vi "CommandParser.vi"(0 "Settings in":T3, 5 "UART_Command":T2, 9 "Cmd_data":u16) -> (4 "Settings out":T3, 6 "UART Reply":T1, 10 "Reply_Data":u16)   [LabVIEW 2013, in "UART_Firmware.lvlib"]
uses:
  UART_Firmware.lvlib
  Settings.ctl
  Parity.ctl
  StopBits.ctl
  UART_Command.ctl
  UART_Response.ctl
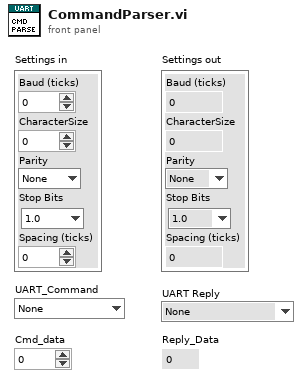
[diagram p1: front panel]
types:
  T1 = typedef "UART_Firmware.lvlib/UART_Response.ctl" = enum8{"None", "Rx", "BaudHighAck", "BaudLowAck", "CharSizeAck", "ParityAck", "StopBitsAck", "SpacingHighAck", "SpacingLowAck", "ParityError", "FrameError"}
  T2 = typedef "UART_Firmware.lvlib/UART_Command.ctl" = enum8{"None", "Tx", "SetBaud_High", "SetBaud_Low", "SetCharLength", "SetParity", "SetStopBits", "SetSpacing_High", "SetSpacing_Low"}
  T3 = typedef "UART_Firmware.lvlib/Settings.ctl" = cluster{"Baud (ticks)":u32, "CharacterSize":u8, "Parity":T4, "Stop Bits":T5, "Spacing (ticks)":u32}
  T4 = typedef "UART_Firmware.lvlib/Parity.ctl" = enum8{"None", "Even", "Odd"}
  T5 = typedef "UART_Firmware.lvlib/StopBits.ctl" = enum8{"1.0", "1.5", "2.0"}
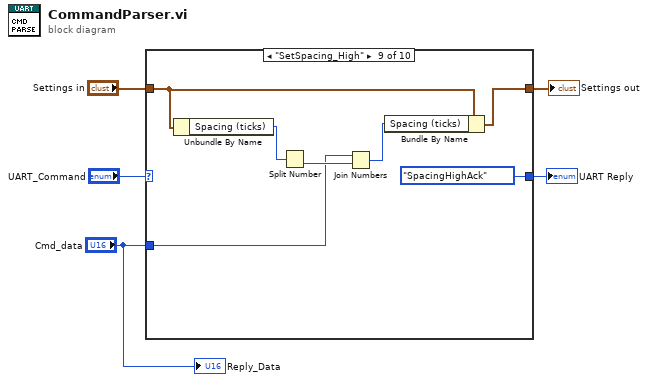
[diagram p0: block diagram]
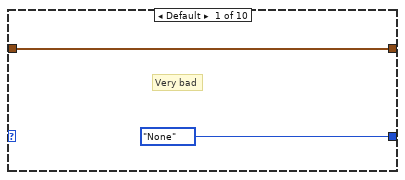
[diagram p2: hidden frame]
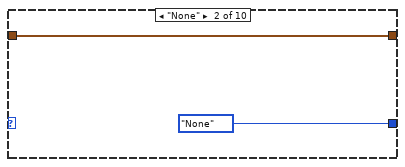
[diagram p3: hidden frame]
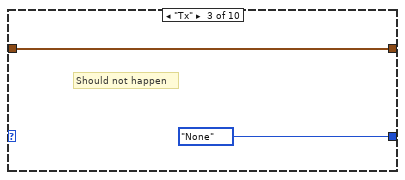
[diagram p4: hidden frame]
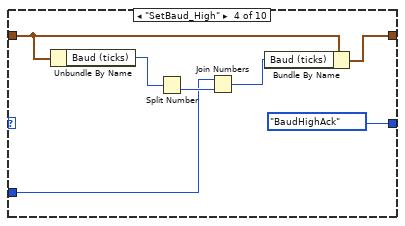
[diagram p5: hidden frame]
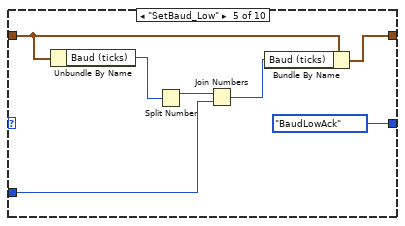
[diagram p6: hidden frame]
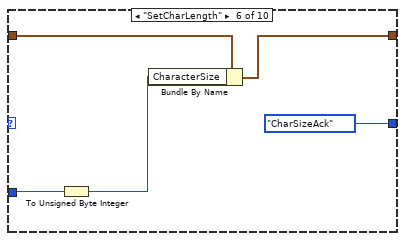
[diagram p7: hidden frame]
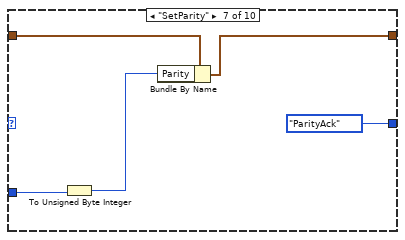
[diagram p8: hidden frame]
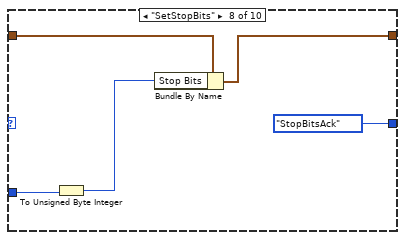
[diagram p9: hidden frame]
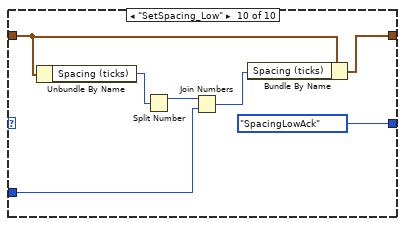
[diagram p10: hidden frame]
diagram:
  n1 = case shown="\"SetSpacing_High\"" "UART_Command" {
    tunnel: "Settings in" -> [w6 w9 w11 w18 w25 w30 w35 w40 w46 w53]
    tunnel: "Cmd_data" -> [_ _ _ w13 w20 w27 w32 w37 w41 w49]
    tunnel: [w6 w9 w11 w16 w23 w29 w34 w39 w47 w54] -> w3
    tunnel: [UART_Response."None" ("UART Reply") UART_Response."None" ("UART Reply") UART_Response."None" ("UART Reply") UART_Response."BaudHighAck" ("UART Reply") UART_Response."BaudLowAck" ("UART Reply") UART_Response."CharSizeAck" ("UART Reply") UART_Response."ParityAck" ("UART Reply") UART_Response."StopBitsAck" ("UART Reply") UART_Response."SpacingHighAck" ("UART Reply") UART_Response."SpacingLowAck" ("UART Reply")] -> w2
    frame Default {
      # "Very bad"
    }
    frame "None" {
    }
    frame "Tx" {
      # "Should not happen"
    }
    frame "SetBaud_High" {
      n2 = Unbundle By Name(w18) -> ("Baud (ticks)"=w15:u32)
      n3 = Split Number(x=w15) -> (lo(x)=w14:u16)  [unwired: 1 out]
      n4 = Join Numbers(hi=w13, lo=w14) -> ((hi.lo)=w12:u32)
      n5 = Bundle By Name(cluster=w18, "Baud (ticks)"=w12) -> (w16:T3)
    }
    frame "SetBaud_Low" {
      n6 = Unbundle By Name(w25) -> ("Baud (ticks)"=w22:u32)
      n7 = Split Number(x=w22) -> (hi(x)=w21:u16)  [unwired: 1 out]
      n8 = Join Numbers(hi=w21, lo=w20) -> ((hi.lo)=w19:u32)
      n9 = Bundle By Name(cluster=w25, "Baud (ticks)"=w19) -> (w23:T3)
    }
    frame "SetCharLength" {
      n10 = To Unsigned Byte Integer(number=w27) -> (unsigned 8bit integer=w26:u8)
      n11 = Bundle By Name(cluster=w30, "CharacterSize"=w26) -> (w29:T3)
    }
    frame "SetParity" {
      n12 = To Unsigned Byte Integer(number=w32) -> (unsigned 8bit integer=w31:u8)
      n13 = Bundle By Name(cluster=w35, "Parity"=w31) -> (w34:T3)
    }
    frame "SetStopBits" {
      n14 = To Unsigned Byte Integer(number=w37) -> (unsigned 8bit integer=w36:u8)
      n15 = Bundle By Name(cluster=w40, "Stop Bits"=w36) -> (w39:T3)
    }
    frame "SetSpacing_High" {
      n16 = Unbundle By Name(w46) -> ("Spacing (ticks)"=w44:u32)
      n17 = Split Number(x=w44) -> (lo(x)=w42:u16)  [unwired: 1 out]
      n18 = Join Numbers(hi=w41, lo=w42) -> ((hi.lo)=w43:u32)
      n19 = Bundle By Name(cluster=w46, "Spacing (ticks)"=w43) -> (w47:T3)
    }
    frame "SetSpacing_Low" {
      n20 = Unbundle By Name(w53) -> ("Spacing (ticks)"=w51:u32)
      n21 = Split Number(x=w51) -> (hi(x)=w50:u16)  [unwired: 1 out]
      n22 = Join Numbers(hi=w50, lo=w49) -> ((hi.lo)=w48:u32)
      n23 = Bundle By Name(cluster=w53, "Spacing (ticks)"=w48) -> (w54:T3)
    }
  }
  "Settings out" <- w3
  "UART Reply" <- w2
  "Reply_Data" <- "Cmd_data"
